vi "Prompt for Step.vi"(8 "error in (no error)":errorcluster, 10 "Subpanel Ref":refnum<vi>, 11 "Image Assertion in":refnum<class "Image Assertion.lvclass">) -> (0 "error out":errorcluster, 3 "Image Assertion out":refnum<class "Image Assertion.lvclass">)   [LabVIEW 2020, in "MacroAssert.lvlib" / "Image Assertion.lvclass"]
doc: "Displays its own window into <B>Subpanel Ref</B> for the user to enter a macro step."
uses:
  Image Assertion.lvclass
  Assertion Step/Assertion Step.lvclass
panel:
  in  "Image Units":u16(ring) items=["Pixels", "Percent"]
  in  "Stop on Fail?":bool
  in  "Comparison Type":u16(ring) items=["Equals", "Does not equal"]
  in  "Left":i16
  in  "Top":i16
  in  "Width":i16
  in  "Height":i16
  in  "Object Name":string
  out "Comparison Value":picture
  out "Subtype Description":string
  in  "Step Subtype":u16(ring) items=["Control Image", "VI Image", "Window Image", "Cursor Icon"]
  # "Press Macro Hotkey to capture\nexpected value"
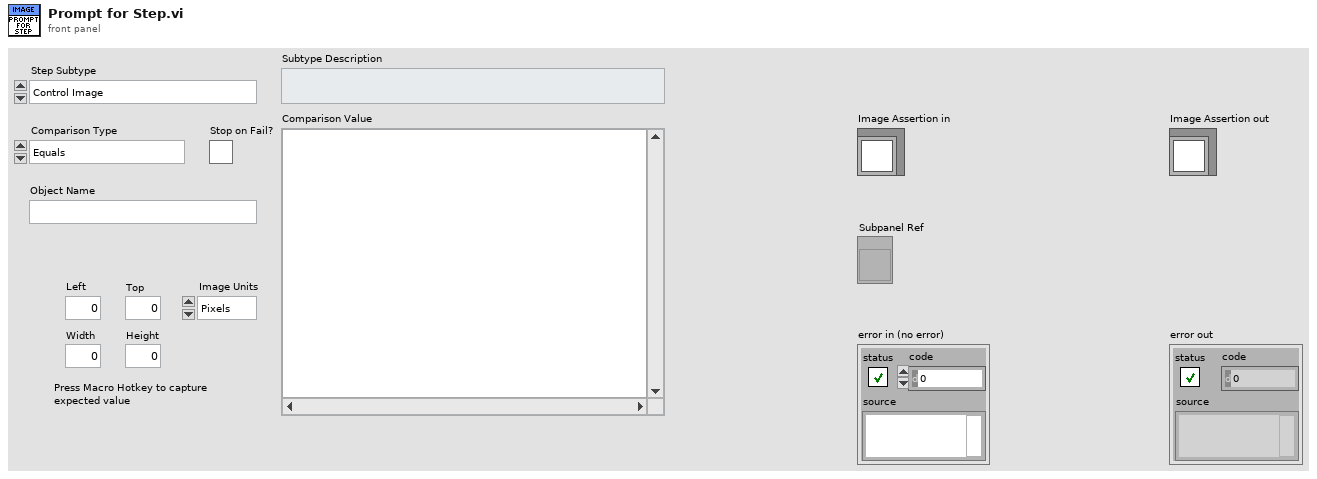
[diagram p1: front panel]
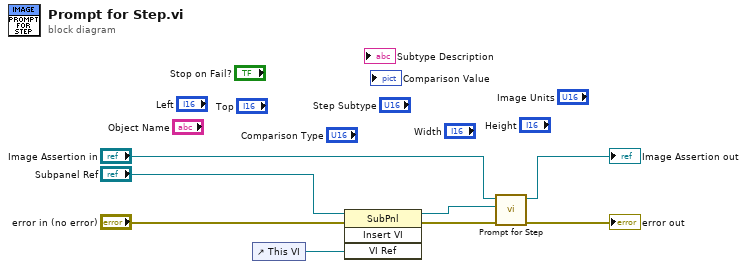
[diagram p0: block diagram]
diagram:
  n1 = control-ref of="This VI"() -> (w6:refnum<vi>)
  n2 = invoke class="SubPnl" method="Insert VI"(reference="Subpanel Ref", error in="error in (no error)", "VI Ref"=w6) -> (reference out=w7:refnum<vi>, error out=w8:errorcluster)  [unwired: 1 in, 2 out]
  n3 = call-parent "Prompt for Step.vi"("error in (no error)"=w8, "Subpanel Ref"=w7, "Step in"="Image Assertion in") -> ("error out"=→"error out":errorcluster, "Step out"=→"Image Assertion out":refnum<class "Image Assertion.lvclass">)  [unwired: 7 in]
